vi "Macro Commit.vi"(8 "error in (no error)":errorcluster, 10 "msg":string, 11 "Git in":refnum<class "Git.lvclass">) -> (0 "error out":errorcluster, 3 "Git out":refnum<class "Git.lvclass">)   [LabVIEW 2019, in "Git.lvclass"]
uses:
  Git.lvclass
  Git.lvclass/Git.ctl
  <vilib>/Hampel Software Engineering/Git API/Git API/GIT-api.lvclass
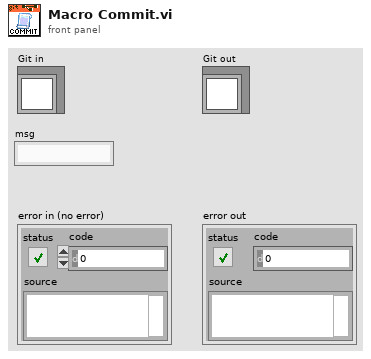
[diagram p1: front panel]
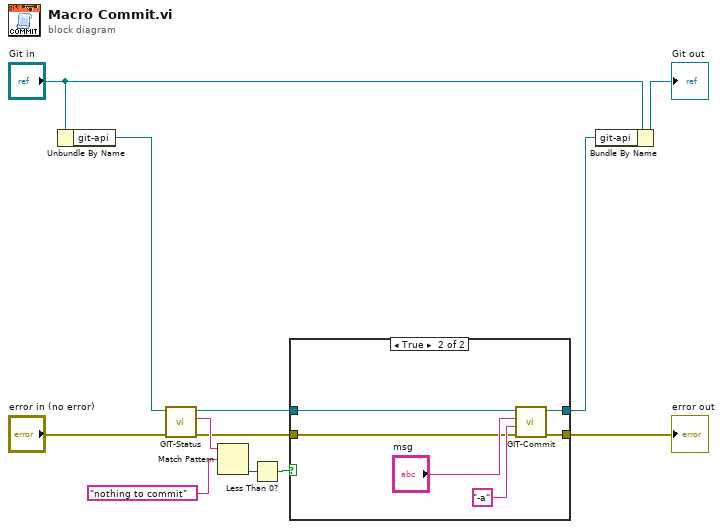
[diagram p0: block diagram]
diagram:
  n1 = Unbundle By Name("Git in") -> ("git-api"=w2:refnum<class "GIT-api.lvclass">)
  n2 = call <vilib>:"GIT-Status.vi"("error in"="error in (no error)", "git-api in"=w2) -> ("error out"=w4:errorcluster, "std out"=w9:string, "git-api out"=w5:refnum<class "GIT-api.lvclass">)  [unwired: 7 in]
  n3 = Match Pattern(string=w9, regular expression="nothing to commit") -> (offset past match=w7:i32)  [unwired: 1 in, 3 out]
  n4 = Less Than 0?(x=w7) -> (x < 0?=w3:bool)
  n5 = case shown="True" w3 {
    tunnel: [w14 w18] -> w10
    tunnel: [w13 w17] -> w6
    tunnel: w5 -> [w14 w16]
    tunnel: w4 -> [w13 w15]
    frame False {
    }
    frame True {
      n6 = call <vilib>:"GIT-Commit.vi"("error in"=w15, "params"="-a", "msg"="msg", "Git-API in"=w16) -> ("error out"=w17:errorcluster, "Git-API out"=w18:refnum<class "GIT-api.lvclass">)  [unwired: 6 in]
    }
  }
  "error out" <- w6
  n7 = Bundle By Name(cluster="Git in", "git-api"=w10) -> (→"Git out":refnum<class "Git.lvclass">)
